vi "EFW Get Product I Ds.vi"(8 "error in (no error)":errorcluster caption="错误输入（无错误）", 11 "pPIDs":i32) -> (0 "error out":errorcluster caption="错误输出", 2 "function return":i32, 3 "pPIDs out":i32)   [LabVIEW 2012, in "EFW_filter.lvlib"]
doc: "EFW_API int EFWGetProductIDs(int* pPIDs);"
uses:
  <userlib>/EFW_filter/EFW_filter.lvlib
  <userlib>/EFW_filter/EFW_filter.dll
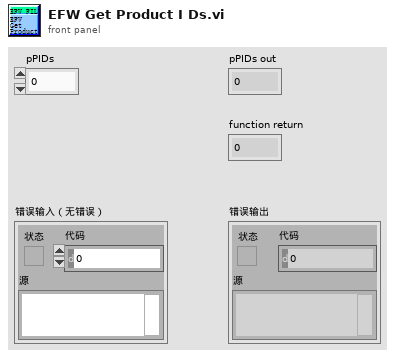
[diagram p1: front panel]
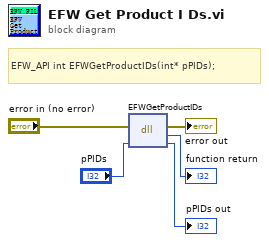
[diagram p0: block diagram]
diagram:
  # "EFW_API int EFWGetProductIDs(int* pPIDs);"
  n1 = dll-call lib="D:/Program Files (x86)/National Instruments/LabVIEW 2012/user.lib/EFW_filter/EFW_filter.*" fn="EFWGetProductIDs"(error in="error in (no error)", "pPIDs"="pPIDs") -> (error out=→"error out":errorcluster, →"function return":i32, "pPIDs"=→"pPIDs out":i32)  [unwired: 2 in, 1 out]
